vi "Measurement.Free.GetPrivateEvents.vi"(8 "error in (no error)":errorcluster, 11 "Measurement.Free":refnum<class "Measurement.Free.lvclass">) -> (0 "error out":errorcluster, 2 "Private Events":T1, 3 "Measurement.Free out":refnum<class "Measurement.Free.lvclass">)   [LabVIEW 2017, in "Measurement.Free.lvclass"]
doc: "---------------------------------------------------------------\nJKI State Machine Objects™\nhttp://jki.net/state-machine-objects/\nCopyright (C) 2005-2015, JKI <info@jki.net>\nALL RIGHTS RESERVEDJKI State Machine Objects (SMO) 1.0.0.4\nJKI - JKI\nCopyright (c) 2015, JKI"
uses:
  Measurement.Free.lvclass
  Typedefs/PrivateEvents--Cluster.ctl
  Typedefs/PrivateEvents--Measurement.Free.SMU.SetVoltage.ctl
  Typedefs/PrivateEvents--Measurement.Free.OPA.SetWavelength.ctl
  Typedefs/PrivateEvents--Measurement.Free.OPA.SetShutterState.ctl
  Measurement.Free.lvclass/Measurement.Free.ctl
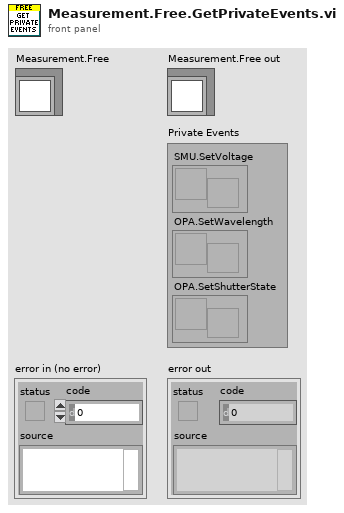
[diagram p1: front panel]
types:
  T1 = typedef "Measurement.Free.lvclass/PrivateEvents--Cluster.ctl" = cluster{"SMU.SetVoltage":refnum<user-event>, "OPA.SetWavelength":refnum<user-event>, "OPA.SetShutterState":refnum<user-event>}
  T2 = typedef "Measurement.Free.lvclass/PrivateData--Ref.ctl" = refnum<data-value>
  T3 = typedef "Measurement.Free.lvclass/PrivateData--Cluster.ctl" = cluster{"Configuration":T4, "Dependencies":T14, "Private Events":T1}
  T4 = typedef "Measurement.Free.lvclass/Configuration--Cluster.ctl" = cluster{"Measurement.Type":enum16{"Free", "I/V Curve", "Wavelength sweeping", "Photocurrent mapping"}, "Hardware":T5}
  T5 = typedef "Measurement.Free.lvclass/Configuration.Hardware--Cluster.ctl" = cluster{"SMU":T6, "LIA":T8, "OPM":T10, "OPA":T12}
  T6 = typedef "Measurement.lvclass/Configuration.SMU--Cluster.ctl" = cluster{"Enable":bool, "SMU Model":string, "Configuration":T7}
  T7 = typedef "SMU.lvclass/Configuration--Cluster.ctl" = cluster{"VISA Resource":string, "Channel":string}
  T8 = typedef "Measurement.lvclass/Configuration.LIA--Cluster.ctl" = cluster{"Enable":bool, "LIA Model":string, "Configuration":T9}
  T9 = typedef "LIA.lvclass/Configuration--Cluster.ctl" = cluster{"VISA Resource":string}
  T10 = typedef "Measurement.lvclass/Configuration.OPM--Cluster.ctl" = cluster{"Enable":bool, "OPM Model":string, "Configuration":T11}
  T11 = typedef "OPM.lvclass/Configuration--Cluster.ctl" = cluster{"VISA Resource":string}
  T12 = typedef "Measurement.lvclass/Configuration.OPA--Cluster.ctl" = cluster{"Enable":bool, "OPA Model":string, "Configuration":T13}
  T13 = typedef "OPA.lvclass/Configuration--Cluster.ctl" = cluster{"Serial Number":string}
  T14 = typedef "Measurement.Free.lvclass/Dependencies--Cluster.ctl" = cluster{"SMU":refnum<class "SMU.lvclass">, "LIA":refnum<class "LIA.lvclass">, "OPM":refnum<class "OPM.lvclass">, "OPA":refnum<class "OPA.lvclass">}
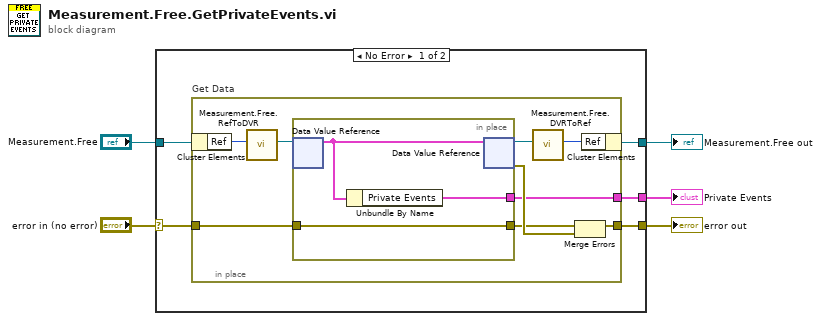
[diagram p0: block diagram]
diagram:
  n1 = case shown="No Error" "error in (no error)" {
    selector: "error in (no error)" -> [w9 w23]
    tunnel: "Measurement.Free" -> [w10 w24]
    tunnel: [w7 w23] -> w4
    tunnel: [w8 w24] -> w3
    tunnel: [w6 _] -> w1
    frame No Error {
      n2 = in-place "Get Data" {
        in-place-border: w9 -> [w19]
        in-place-border: [w16] -> w7
        in-place-border: [w15] -> w6
        n3 = in-place-cluster #1(w10) -> ("Ref"=w14:u32)
        n4 = call "Measurement.Free.RefToDVR.vi"("Ref"=w14) -> ("Ref"=w12:T2)  [unwired: 10 in]
        n5 = in-place {
          in-place-border: w19 -> [w21]
          in-place-border: [w21] -> w17
          in-place-border: [w20] -> w15
          n6 = in-place-dvr #2(w12) -> (w22:T3)  [unwired: 1 out]
          n7 = Unbundle By Name(w22) -> ("Private Events"=w20:T1)
          n8 = in-place-dvr #2(w22) -> (w13:T2, w18:errorcluster)
        }
        n9 = call "Measurement.Free.DVRToRef.vi"("Ref"=w13) -> ("Ref"=w11:u32)  [unwired: 10 in]
        n10 = Merge Errors(w17, w18) -> (w16:errorcluster)
        n11 = in-place-cluster #1("Ref"=w11) -> (w8:refnum<class "Measurement.Free.lvclass">)
      }
    }
    frame Error {
    }
  }
  "error out" <- w4
  "Measurement.Free out" <- w3
  "Private Events" <- w1
